vi "Execute Create New DQMH Message Case.vi"(6 "Mouse Position":T1, 8 "User VI Ref":refnum<vi>, 9 "Menu Item Tag Suffix":string, 10 "Remaining Items":refnum<vi>[](array[refnum]), 11 "Affected Items":T2) -> (0 "Fail transaction?":bool)   [LabVIEW 2025]
doc: "This VI is part of a plug-in for modifying the LabVIEW shortcut menus. This is the execute VI which is called when the shortcut menu is chosen by the user. It performs the action of the selected menu item."
uses:
  Create New DQMH Message Case.ctl
  <vilib>/Utility/miscctls.llb/LVPositionTypeDef.ctl
  <vilib>/Utility/traverseref.llb/TRef TravTarget.ctl
panel:
  out "error out":errorcluster
  # "All controls on this panel except \"Affected Items\" have been locked to prevent accidental edits. Changing the control names or types, other than the elements of the \"Affected Items\" cluster will make the VI unusable as a menu plugin.\n\nSee Context Help for each control for details about its use."
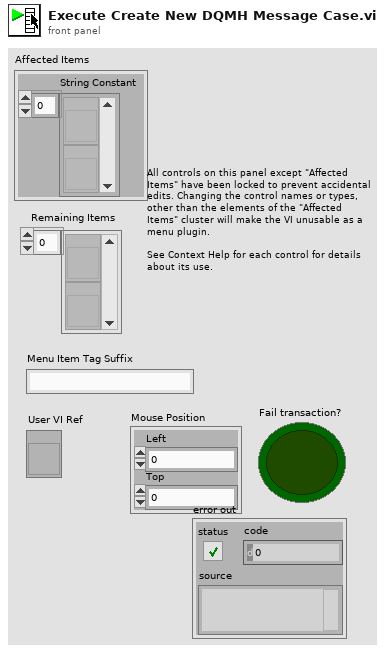
[diagram p1: front panel]
types:
  T1 = typedef "LVPositionTypeDef.ctl" = cluster{"Left":i32, "Top":i32}
  T2 = typedef "Create New DQMH Message Case.ctl" = cluster{"String Constant":refnum<vi>[]}
  T3 = typedef "TRef TravTarget.ctl" = enum16{"FP", "BD", "Other"}
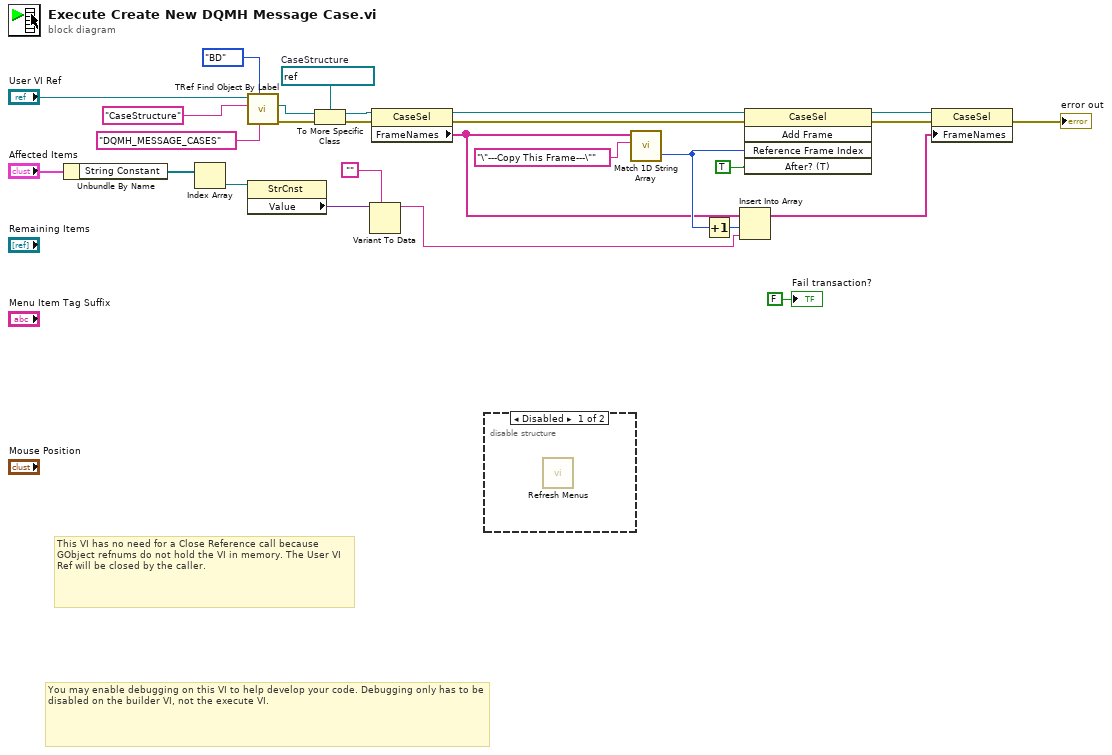
[diagram p0: block diagram]
diagram:
  w18 = refnum<vi> refnum  # CaseStructure
  # "You may enable debugging on this VI to help develop your code. Debugging only has to be disabled on the builder VI, not the execute VI."
  # "This VI has no need for a Close Reference call because GObject refnums do not hold the VI in memory. The User VI Ref will be closed by the caller."
  n1 = Unbundle By Name("Affected Items") -> ("String Constant"=w26:refnum<vi>[])
  n2 = Index Array(array=w26) -> (element=w25:refnum<vi>)  [unwired: 1 in]
  n3 = call <vilib>:"TRef Find Object By Label.vi"("Label"="DQMH_MESSAGE_CASES", "Traverse Target"=TRef_TravTarget."BD", "Class Name"="CaseStructure", "VI Ref"="User VI Ref") -> ("error out"=w2:errorcluster, "Found Obj Ref"=w1:refnum<vi>)  [unwired: 4 in, 2 out]
  n4 = property class="StrCnst"(reference=w25) -> ("Value"=w24:variant)  [unwired: 1 in, 2 out]
  n5 = To More Specific Class(target class=w18, reference=w1, error in=w2) -> (specific class reference=w19:refnum<vi>, error out=w3:errorcluster)
  n6 = Variant To Data(type="", Variant=w24) -> (data=w6:string)  [unwired: 1 in, 1 out]
  n7 = property class="CaseSel"(reference=w19, error in=w3) -> (reference out=w17:refnum<vi>, error out=w16:errorcluster, "FrameNames"=w4:string[])
  n8 = disable-structure shown="Disabled" {
    frame Disabled {
      n9 = call <resource>:"Refresh Menus.vi"() -> ()  [unwired: 12 in]
    }
    frame Enabled {
    }
  }
  n10 = call <vilib>:"Match 1D String Array.vi"("Pattern"="\"---Copy This Frame---\"", "Strings"=w4) -> ("index of element"=w13:i32)  [unwired: 2 in, 1 out]
  n11 = Increment(x=w13) -> (x+1=w12:i32)
  n12 = Insert Into Array(array=w4, index=w12, new element=w6) -> (w5:string[])
  n13 = invoke class="CaseSel" method="Add Frame"(reference=w17, error in=w16, "Reference Frame Index"=w13, "After? (T)"=TRUE) -> (reference out=w11:refnum<vi>, error out=w10:errorcluster)  [unwired: 1 in, 3 out]
  n14 = property class="CaseSel"(reference=w11, error in=w10, "FrameNames"=w5) -> (error out=→"error out":errorcluster)  [unwired: 1 out]
  "Fail transaction?" <- FALSE ("Fail transaction?")
